vi "AVGof3.vi"(1 "Input c":dbl, 2 "Input b":dbl, 3 "Input a":dbl) -> (0 "Average of a,b,c":dbl)   [LabVIEW 2019]
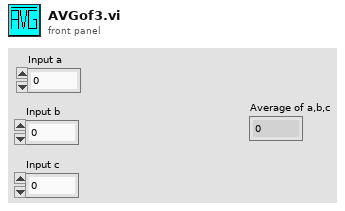
[diagram p1: front panel]
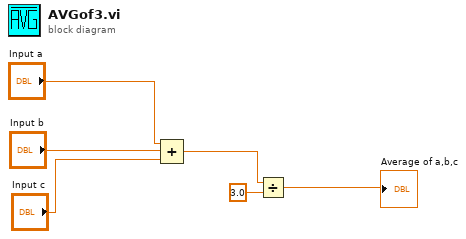
[diagram p0: block diagram]
diagram:
  n1 = Compound Arithmetic op=ADD("Input a", "Input b", "Input c") -> (w3:dbl)
  n2 = Divide(x=w3, y=3.0) -> (x/y=→"Average of a,b,c":dbl)
